vi "AlliGator Overlays Phasor Ratio or Derived Quantity on Source Image v3.vi"(7 "Image Color Scale Information":T2, 8 "Error In":errorcluster, 10 "Source Image Display":T1, 11 "AlliGator IV DVR in":refnum<data-value>) -> (0 "Error Out":errorcluster, 1 "# Overlay Pixels":i32, 2 "Source Image Display out":T1, 3 "AlliGator IV DVR out":refnum<data-value>)   [LabVIEW 2021, in "AlliGator Phasor Ratio.lvlib"]
doc: "Computes and overlays the phasor ratio map (or map of a derived quantity) on the Source Image."
uses:
  AlliGator Phasor Ratio.lvlib
  <vilib>/vision/Image Controls.llb/IMAQ Image.ctl
  AlliGator Internal Variables v2.ctl
  AlliGator Gate Image Set.ctl
  AlliGator FLI Dataset Type.ctl
  AlliGator Data Series Type.ctl
  AlliGator Dataset Channel.ctl
  AlliGator Gate Arithmetic.ctl
  AlliGator Displayed Image.ctl
  Image/Named ROI Description.ctl
  AlliGator Decay Metadata v3.ctl
  AlliGator Decay Background Subtraction Info.ctl
  AlliGator Baseline Subtraction Method.ctl
  Graphs/XY Graph/XY Graph Plot Shift Parameters.ctl
  Graphs/XY Graph/XY Graph Plot Shift Method.ctl
  AlliGator Decay Extrapolation Parameters.ctl
  Phasor/Calibration Phasor (m, phi).ctl
  Phasor/Phasor Reference Series.ctl
  Phasor/Phasor Calibration Map v2.ctl
  Phasor/Phasor (g, s).ctl
  AlliGator Raw Phasor Plot Data v4.ctl
  Phasor/Phasor Standard Deviation Options.ctl
  AlliGator Phasor Multi-Harmonic Data.ctl
  Phasor/Phasor Harmonic Data.ctl
  AlliGator Decay Fit Options & Parameters v2.ctl
  Fits/IRF(X)PSED/Decay Fit Options v2.ctl
  Fits/Decay Convolution/Decay Model.ctl
  Fits/Residual Type.ctl
  Fits/IRF(X)PSED/Fit Weights Type.ctl
  Fits/Non-linear Fitting Method v2.ctl
  Fits/Fit Calculation Method.ctl
  Fits/Non-linear Fitting Algorithm.ctl
  AlliGator Decay Fit Parameter Constraints 2.ctl
  Fits/IRF(X)PSED/Decay Fit Parameters In List.ctl
  Fits/IRF(X)PSED/MLE Baseline Offset Type.ctl
  AlliGator Decay Preprocessing Parameters.ctl
  Fits/IRF(X)PSED/Decay Fit Parameters & Derived Quantities List.ctl
  AlliGator Parameter Maps Data.ctl
  Image/Image Color Scale Information.ctl
  AlliGator Settings List.ctl
  Palette/Image Palette Information.ctl
  Image/Image Display Palette Type.ctl
  AlliGator Variables List.ctl
  AlliGator Phasor Ratio Data.ctl
  AlliGator Phasor Ratio Color-Coded Quantity.ctl
  Phasor/Phasor Ratio Type.ctl
  AlliGator Partial Data Information.ctl
  Variant/Variant to Data/Variant to DBL.vi
  Variant/Variant to Data/Variant to Boolean.vi
  Variant/Variant to Data/Variant to String.vi
  Image/Image Get Pixel Color.vi
  Image/Adjust Pixel Overlay Brightness.vi
  <vilib>/vision/NI_Vision_Development_Module.lvlib
  AlliGator Settings.lvlib
  Variant/Variant to Data/Variant to Data.lvlib
  Image/Image.lvlib
  Palette/Palette.lvlib
  AlliGator Globals, Variables & Constants.lvlib
  Time/Time.lvlib
  Error/Error.lvlib
  Phasor/Phasor.lvlib
  Utilities/Utilities.lvlib
  AlliGator Phasor Plot.lvlib
  AlliGator Decay Preprocessing.lvlib
  Graphs/XY Graph/XY Graph Add-Ons.lvlib
  AlliGator Phasor Graph.lvlib
  AlliGator Files.lvlib
  AlliGator Source Image.lvlib
  AlliGator Internal Variables.lvlib
  Fits/Fits.lvlib
  AlliGator Decay Fit.lvlib
  AlliGator Decay Fit Parameter Map.lvlib
  AlliGator Dual-Channel Datasets.lvlib
panel:
  out "Overlay Copy (s)":dbl
  out "Overlay Erase (s)":dbl
  out "Overlay Compute (s)":dbl
  # "see the AlliGator License on the block diagram (Ctrl+E or Window:Show Block Diagram)"
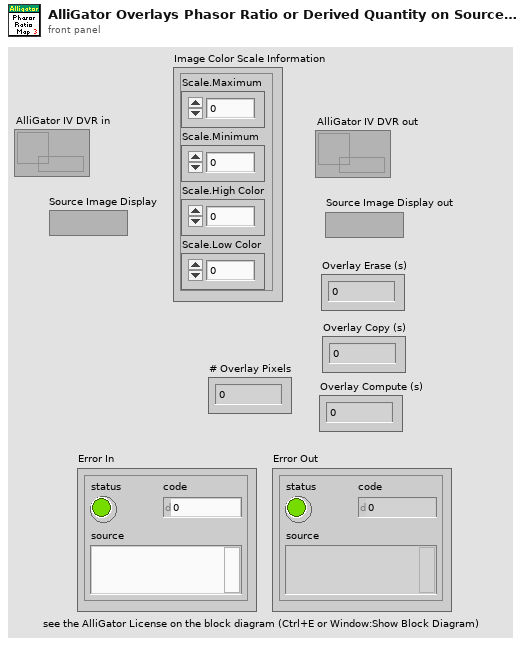
[diagram p1: front panel]
types:
  T1 = typedef "IMAQ Image.ctl" = refnum<image>
  T2 = typedef "Image.lvlib/Image Color Scale Information.ctl" = cluster{"Scale.Maximum":dbl, "Scale.Minimum":dbl, "Scale.High Color":u32, "Scale.Low Color":u32}
  T3 = typedef "AlliGator Settings.lvlib/AlliGator Settings List.ctl" = enum16{"GUI:Visible Settings Tab", "GUI:Last Run Version", "Source Image:Use Image Histogram for Contrast", "Source Image:Low Count Pixels Rejection Options", "Source Image:High Count Pixels Rejection Options", "Source Image:Use Image Brightness", "Source Image:Blend Overlay with Image Background", "Source Image:Use Fixed ROI Diameter", "Source Image:ROI Diameter", "Source Image:ROI Center Color", "Source Image:Peak Threshold", "Source Image:Intensity Threshold", "Source Image:Image Binning Options", "Source Image:Image Smoothing Options", "Source Image:Image Histogram Active", "Source Image:Invert Binary Mask", "Source Image:Hot Pixel Removal", "Source Image:Overlay Analyzed ROI Center", "Source Image:Auto-Adjust Contrast", "Source Image:Histogram Lower Percentile", "Source Image:Histogram Upper Percentile", "Source Image:Save Source Image", "Source Image:Scale Bar Options", "Source Image:Image Resolution (Pixel Size)", "Source Image:Flatfield Correction", "Source Image:Show Dead Left Columns Correction", "Source Image:Dead Left Columns Correction", "Source Image:Image Pre-Processing Operations Order", "Data Information:Gate Width", "Data Information:Nanotime Gate Separation", "Data Information:Macrotime Gate Separation", "Data Information:Gate Step", "Data Information:# Gates", "Data Information:Gate Image Exposure", "Data Information:Gate Image Integration", "Data Information:Gates to Skip", "Data Information:Gates to Keep", "Data Information:Define Gates to", "Data Information:Channel Name", "Data Information:Available Channel Names", "Data Information:Channel Arithmetic", "Data Information:Background File Subtraction", "Data Information:Background File", "Data Information:Background Scaling Factor", "Data Information:Background Pile-up Correction", "Data Information:Background Pixel Well Capacity", "Data Information:Laser Period", "Data Information:SYNC Period", "Data Information:Pile-up Correction", "Data Information:Pixel Well Capacity", "Data Information:Dataset Scaling Factor", "Fluorescence Decay_Decay Pre-Processing:Reverse Gates", "Fluorescence Decay_Decay Pre-Processing:Verbose Decay Pre-Processing", "Fluorescence Decay_Decay Pre-Processing:Use Decay Pre-Processing", "Fluorescence Decay_Decay Pre-Processing:Background Subtraction", "Fluorescence Decay_Decay Pre-Processing:Background Definition Range", "Fluorescence Decay_Decay Pre-Processing:Baseline Subtraction Method", "Fluorescence Decay_Decay Pre-Processing:Decay Pre-Processing Operations Order", "Fluorescence Decay_Decay Pre-Processing:Smoothing Parameter", "Fluorescence Decay_Decay Pre-Processing:Shift Decay", "Fluorescence Decay_Decay Pre-Processing:Decay Shift Parameters", "Fluorescence Decay_Decay Pre-Processing:Fold Decay", "Fluorescence Decay_Decay Pre-Processing:# Folds", "Fluorescence Decay_Decay Pre-Processing:1-Normalize Decay", "Fluorescence Decay_Decay Pre-Processing:[0-1]-Normalize Decay", "Fluorescence Decay_Decay Pre-Processing:Smoothen Decay", "Fluorescence Decay_Decay Pre-Processing:Extrapolate Decay", "Fluorescence Decay_Decay Pre-Processing:Use Periodicity", "Fluorescence Decay_Decay Pre-Processing:Use Cursors", "Fluorescence Decay_Decay Pre-Processing:Tail Fraction", "Fluorescence Decay_Decay Pre-Processing:Head Fraction", "Fluorescence Decay_Decay Pre-Processing:Additional Points", "Fluorescence Decay_Decay Pre-Processing:Straighten Decay", "Fluorescence Decay_Decay Pre-Processing:Constant Background", "Fluorescence Decay_Decay Pre-Processing:Pixel-Normalize Decay", "Fluorescence Decay_Advanced Analysis:Extract IRF instead of Decay", "Fluorescence Decay_Advanced Analysis:IRF Extraction Options", "Fluorescence Decay_Advanced Analysis:IRF Optimization Options", "Fluorescence Decay_Advanced Analysis:Square Pulse Options", "Fluorescence Decay_Advanced Analysis:IRF Order", "Fluorescence Decay_Advanced Analysis:IRF Time Constants", "Fluorescence Decay_Advanced Analysis:Wavelet Analysis Options", "Fluorescence Decay_Advanced Analysis:Average Lifetime Options", "Fluorescence Decay_Fit Options:Fit Options", "Fluorescence Decay_Fit Options:Use Legacy Fitting Approach", "Fluorescence Decay_Fit Options:Use Data Information Laser Period", "Fluorescence Decay_Fit Parameters:Displayed Fit Parameters", "Fluorescence Decay_Fit Parameters:Fit Parameter Constraints", "Fluorescence Decay_Fit Parameters:Export Tabulated Results", "Fluorescence Decay_Fit Parameters:MLE Baseline Offset Type", "Fluorescence Decay_Fit Parameters:MLE Baseline Offset", "Fluorescence Decay_Fit Parameters:Guess Parameter Names", "Fluorescence Decay_Fit Parameters:Guess Parameter Values", "Fluorescence Decay_Fit Parameters:Guess Parameters Options", "Fluorescence Decay_Styles:Show Last Decay Only", "Fluorescence Decay_Styles:Decay Graph Color Array", "Fluorescence Decay:Decay Graph Active", "Fluorescence Decay Statistics:Min Peak Value", "Fluorescence Decay Statistics:Reject Low Decay Peak Pixels", "Fluorescence Decay Statistics:Reject High Decay Peak Pixels", "Fluorescence Decay Statistics:Max Peak Value", "Time Traces:Use File Timestamp", "Time Traces:Time Step", "Time Traces:Use Intensity Correction File", "Time Traces:Intensity Correction File", "Phasor Plot:Phasor Plot Smoothing Options", "Phasor Plot:Phasor Plot Size", "Phasor Plot:Phasor Plot Graphics Options", "Phasor Plot:Cumulative Phasor Plot", "Phasor Plot:Use Phasor Brightness", "Phasor Plot:Blend Overlay with Phasor Background", "Phasor Plot:Save Phasor Plot", "Phasor Plot:Show References", "Phasor Plot:Phasor Ratio Decay Range", "Phasor Plot:Exponential Fading", "Phasor Plot:Phasor Ratio Reference Colors", "Phasor Plot:Reference Radius", "Phasor Plot:Show Color Map Vertices", "Phasor Plot:Phasor Plot Active", "Phasor Plot:Phasor Ratio Color Map Type", "Phasor Plot:Phasor Ratio Color Map", "Phasor Plot:Phasor Ratio Display Range", "Phasor Plot:Selected Image ROI(s)", "Phasor Plot:All Image ROIs", "Phasor Plot:Selected Phasor Plot ROI(s)", "Phasor Plot:All Phasor Plot ROIs", "Phasor Plot:Phasor Ratio Color-Coded Quantity", "Phasor Plot:Store Phasor Harmonics", "Phasor Plot:Draw Reference Segment", "Phasor Plot:User-Defined Quantity", "Phasor Graph:Phasor Frequency", "Phasor Graph:Phasor Ratio Type", "Phasor Graph:Pixel-level Phasor Computation", "Phasor Graph:Save Phasor Graph", "Phasor Graph:Phasor Graph Active", "Phasor Graph:Phasor SDV Options", "Phasor Calibration:Use Backup Calibration if needed", "Phasor Graph:Define Shortest Lifetime as", "Phasor Calibration:Backup Calibration Type", "Phasor Calibration:Calibration Type", "Phasor Calibration:Calibration Lifetime", "Phasor Calibration:Calibration Map Algorithm", "Single-Exponential Phasor Locus (SEPL):Gate Parameters", "Single-Exponential Phasor Locus (SEPL):User-defined Gate", "Single-Exponential Phasor Locus (SEPL):User-defined IRF", "Single-Exponential Phasor Locus (SEPL):Phasor Parameters", "Single-Exponential Phasor Locus (SEPL):Decay & IRF Parameters", "Single-Exponential Phasor Locus (SEPL):Display Parameters", "Lifetime Analysis:Decay Analysis Parameters", "Lifetime Analysis:Lifetime Map Active", "Plugins:Python Settings", "Miscellaneous:Verbose Mode", "Miscellaneous:Beep after Script", "Miscellaneous:Saved Image File Format", "Miscellaneous:Exported Gate Image Settings", "Miscellaneous:Include Loading in Timing", "Miscellaneous:Verbose Settings Mode", "Miscellaneous:Histogram Options", "Miscellaneous:Beep on Error", "Miscellaneous:# Logical Processors Used", "Miscellaneous:ROI Description Max Characters", "Miscellaneous:Verbose Error Mode", "Miscellaneous:Transparent Mask Color"}
  T4 = typedef "AlliGator Settings.lvlib/AlliGator Partial Data Information.ctl" = cluster{"Laser Period":dbl[unit], "SYNC Period":dbl[unit], "# Gates":u32, "Gate Separation":dbl[unit]}
  T5 = typedef "Phasor.lvlib/Phasor Ratio Type.ctl" = enum32{"Intensity-weighted", "Amplitude-weighted"}
  T6 = typedef "AlliGator Phasor Ratio.lvlib/AlliGator Phasor Ratio Color-Coded Quantity.ctl" = enum16{"Phasor Ratio (f1 or a1)", "Average Lifetime (<tau>_i or <tau>_a))", "User-Defined Quantity"}
  T7 = typedef "AlliGator Phasor Ratio.lvlib/AlliGator Phasor Ratio Data.ctl" = cluster{"Complex Phasor":csg, "Phasor Ratio":sgl, "z_1":csg, "z_2":csg, "Mapped Quantity":sgl}
  T8 = typedef "AlliGator Globals, Variables & Constants.lvlib/AlliGator Variables List.ctl" = enum16{"---- GUI ----", "GUI:Initialization Status", "GUI:State Indicators Refnum", "GUI:Original AlliGator Menu Items", "GUI:Current Action Loop State", "GUI:Script in progress", "GUI:Playback", "GUI:Loop Playback", "GUI:Search ROI Used", "GUI:Search ROI", "Decay Graph Max Legend Size", "Intensity Graph Max Legend Size", "Decay Statistics Graph Max Legend Size", "Phasor Graph Max Legend Size", "Phasor Ratio Graph Max Legend Size", "Lifetime Graph Max Legend Size", "---- Files ----", "Files:Export Dataset Frames as Individual Files", "Files:Show Batch Export Help Balloons", "Files:Frames in Dataset", "Files:ptu File Frame Start Indices", "Files:Current Frame in Dataset", "Files:Current Frame Timestamp", "Files:Dataset Loaded", "Files:Dataset Metadata", "Files:Dataset Channel", "Files:Dataset Data Description", "Files:Background Dataset Metadata", "Files:Background Dataset Channel", "Files:Background Dataset Data Description", "Files:Background File Subtraction", "Files:Background File Path", "Files:Background File Pile-up Correction", "Files:Background File Pixel Well Capacity", "Files:Background File Scaling Factor", "Files:Current Dataset Load Settings", "Files:Dataset Path", "Files:ICCD-specific Information", "Files:Macrotime Gate Separation", "------ Python Plugins ------", "Python Plugins:Information", "Python Plugins:Python Session", "Python Plugins:Valid Python Session?", "---- Source Image ----", "Source Image:ROIs", "Source Image:Current ROI", "Source Image:ROI Event Refnum", "X_Source Image Display Range", "X_Source Image Palette Information", "X_Type of Displayed Image", "X_Time Gate Slider", "Source Image:Palette List", "Source Image:Scale", "Source Image:ROI Overlay Color", "Source Image:Overlay to Erase", "Source Image:Is Displayed Image Accumulated", "Source Image:White Light Image Modified", "Source Image:Mask Image Modified", "---- Image Profile Window ----", "Image Profile:Overlay ROI in Source Image", "Image Profile:Window Event Refnum", "Image Profile:IntensityType", "Image Profile:Intensity Average Type", "Image Profile:Intensity-weighted SDV", "Image Profile:Box Profile Type", "Image Profile:Window Open", "Image Profile:Plotted Fit Parameter", "------ Phasor Graph -------", "Phasor Graph:Show Line", "---- Phasor Plot ---", "Phasor Plot:Parameters Changed", "Phasor Plot:FLI Dataset Modified since last Calculation", "Phasor Harmonics Data", "Selected Phasor Harmonics", "Phasor Harmonic Manager Event Refnum", "Phasor Plot:ROIs", "Phasor Plot:Current ROI", "Phasor Plot:ROI Event Refnum", "Phasor Plot:Image Reference Points", "Phasor Plot:Computed", "Phasor Plot:Palette Information", "Phasor Plot:Palette List", "Phasor Plot:Phasor Ratio Palette Information", "Phasor Plot:Phasor Ratio Palette List", "Phasor Plot:Image Scale", "Phasor Plot:Image Overlay to Erase", "Phasor Plot:Image Elements to Update", "Phasor Plot:Current Calculation Parameters", "Phasor Plot:Current Calibration Options", "Phasor Plot:Reset Cumulated Phasor Plot", "Phasor Plot:Reference 1", "Phasor Plot:Lifetime Reference 1", "Phasor Plot:Reference 1 Frequency", "Phasor Plot:Reference 2", "Phasor Plot:Lifetime Reference 2", "Phasor Plot:Reference 2 Frequency", "---- Decay Analysis ----", "Number of Selected Decays to Fit", "LS Fit Results", "LAR Fit Results", "BS Fit Results", "Last Decay Max - Min", "Best Fit Parameters", "Best Fit Parameter Names", "Actual Size X", "Actual Size Y", "Binning X", "Binning Y", "Actual # Gates", "Dataset Number", "Gates to...", "Gates Skipped", "Gates to keep", "Gate Step", "Gate Separation", "Reversed Gates", "Pile-up Correction", "Pixel Well Capacity", "Background Subtracted", "Background Subtraction Method", "Background Definition Range", "Background File (deprecated)", "Number of Dataset Accumulated", "Array of Accumulated Dataset Paths", "Do Averaged Datasets", "Destination File Path", "Process Plot Target", "Use 1/D as Phasor Frequency", "---- Decay Fit Parameter Map -----", "Decay Fit Parameter Map:Palette Information", "Decay Fit Parameter Map:Palette List", "------- Local Decay Window ---------", "Local Decay Graph Window:Event Refnum", "Local Decay Graph Window:Use normalized IRF for convolution", "----- Miscellaneous ----", "Misc:Skippable Dialog Windows Status"}
  T9 = typedef "Palette.lvlib/Image Palette Information.ctl" = cluster{"Palette Name [# Colors,int?,inv?]":string, "Palette Type":T10, "Palette Colors":u32[], "Interpolate?":bool}
  T10 = typedef "Image.lvlib/Image Display Palette Type.ctl" = u32
  T11 = enum32{"Interpolate Reference Colors", "Use Custom Map"}
  T12 = cluster{"Reference 1":u32, "Reference 2":u32, "Boundary":u32}
  T13 = typedef "Phasor.lvlib/Phasor (g, s).ctl" = cluster{"g":dbl, "s":dbl}
  T14 = typedef "AlliGator Internal Variables.lvlib/AlliGator Internal Variables v2.ctl" = cluster{"Displayed Image":T1, "White Light Image":T1, "Mask Image":T1, "ROI Mask Image":T1, "Current Dataset Images 1":T15, "Background Dataset Images 1":T15, "Current Dataset Images 2":T15, "Background Dataset Images 2":T15, "Current Dataset Arithmetic Images":T15, "Accumulated Dataset Images 1":T15, "Accumulated Dataset Images 2":T15, "Accumulated Dataset Arithmetic Images":T15, "Phasor Plot Image":T1, "Decay Fit Parameter Map Image":T1, "Single Data Point Path":path, "White Light Image Path":path, "Mask Image Path":path, "Time-Series Folder":path, "[Time-Series Paths]":path[], "Current Dataset":i32, "Single Dataset Type":T16, "Current Folder":string, "AlliGator Data Series Type":T17, "# Datasets":i32, "Dual-Channel Dataset":bool, "Selected Channel Name":string, "Dataset Channel":T18, "Channel Arithmetic":T19, "Dual-Channel Background Dataset":bool, "Background Channel":T18, "Dual-Channel Accumulated Dataset":bool, "Start Time":dbl, "[Time-Series Timestamps]":dbl[], "[Intensity Corrections]":dbl[], "Time Series Script":bool, "Type of Displayed Image":T20, "Gate Image Slide":u16, "# Gates":i32, "ROIs":T21[], "ROI Decay":cluster{"t Array":dbl[], "I Array":dbl[]}, "Valid Decay":bool, "Decay  Metadata":T23, "Reference Decay Plot Name":string, "Reference Decay":cluster{"t Array":dbl[], "I Array":dbl[]}, "Decay Shift Plot":cluster{"Time Stamps":dbl[], "Decay Shifts":dbl[]}, "[Decays Max Values]":sgl[], "[Decays Min Values]":sgl[], "Calibration Phasor":T29, "Calibration Phasor Series":T30, "Phasor Calibration Map":T31, "Calibration Map MD5 Digest":string, "Last Raw Phasor":T13, "Last Calibrated Phasor":T13, "Last Calibrated Phasor SDV":T13, "Phasor Graph:Phasor Plot":cluster{"g Array":dbl[], "s Array":dbl[]}, "Phasor Graph:Phasor SDV Plot":cluster{"g Array":dbl[], "s Array":dbl[]}, "[Phasor Graph:Raw Phasor Plots]":T32[], "Phasor Plot locked to Ref 1":i32, "[Phasor Plot(s) locked to Ref 1]":i32[], "[Phasor Plot(s) locked to Ref 2]":i32[], "[Pixel Phasors]":T13[], "[[Sum Image]]":dbl[][], "[[CSG Phasors]]":csg[][], "[[Valid Pixel?]]":bool[][], "I/m/phi Dataset":cluster{"I/m/phi Dataset?":bool, "Base Frequency":dbl[unit], "Harmonic Orders":u8[]}, "Multi Phasor Plot Data":T34, "Decay Fit Options & Parameters":T36, "Fit Options: Decay Preprocessing Parameters":T47, "Fit Options: Reference Decay":cluster{"t Array":dbl[], "I Array":dbl[]}, "Is Full Image Parameters Map":bool, "Is Single-Pixels Parameters Map":bool, "NLSF Parameters Map X Resolution":i32, "NLSF Parameters Map Y Resolution":i32, "[Single Decay Fit Parameters]":dbl[], "Fit Model":T38, "[[Multiple Decays Fit Parameters]]":dbl[][], "[[Multiple Decays Fit Parameter SDVs]]":dbl[][], "[[IRFs]]":dbl[][], "IRF Array Time Axis":dbl[], "Decay Array Time Axis":dbl[], "[Decay Fit Parameter Names]":T48[], "[[Phasor Ratios]]":dbl[][], "[[Average Lifetimes]]":dbl[][], "Amplitude Weighted Average Lifetime":bool, "[Decay Sum]":dbl[], "Parameter Maps":T49[], "[[User-defined Quantities]]":dbl[][], "User-defined Quantity":string}
  T15 = typedef "AlliGator Internal Variables.lvlib/AlliGator Gate Image Set.ctl" = cluster{"SGL Image Max":T1, "SGL Image Sum":T1, "SGL Gate Images":T1[], "SGL Image Min":T1}
  T16 = typedef "AlliGator Files.lvlib/AlliGator FLI Dataset Type.ctl" = enum16{"HDF5 FLI Dataset", "Gate Image Folder", ".sdt FLI Dataset (Becker & Hickl)", ".ptu FLI Dataset (PicoQuant)", "SS1 FLI Dataset", "SS2 FLI Dataset", "I/m/phi Dataset", ".bin FLI Dataset (PicoQuant Binned)", ".bin FLI Dataset (Piccolo Binned)"}
  T17 = typedef "AlliGator Files.lvlib/AlliGator Data Series Type.ctl" = enum16{"Not a Supported Series", "Gate Images Folder Series", "SwissSPAD 2 Dataset Series", "B&H FLI Dataset Series", "PicoQuant PTU FLI Dataset Series", "PicoQuant BIN FLI Dataset Series", "Piccolo hist BIN FLI Dataset Series", "HDF5 FLI Dataset Series"}
  T18 = typedef "AlliGator Dual-Channel Datasets.lvlib/AlliGator Dataset Channel.ctl" = enum16{"G2", "INT"}
  T19 = typedef "AlliGator Settings.lvlib/AlliGator Gate Arithmetic.ctl" = enum16{"None", "INT-G2", "G2/INT*<INT>", "(1 - G2/INT)*<INT>"}
  T20 = typedef "AlliGator Source Image.lvlib/AlliGator Displayed Image.ctl" = enum16{"Single Gate", "Sum of All Gates", "Max of All Gates", "Min of All Gates", "-", "White Ligth Image", "Mask Image"}
  T21 = typedef "Image.lvlib/Named ROI Description.ctl" = cluster{"ROI Descriptor":T22, "ROI Name":string, "Overlay Color":u32}
  T22 = typedef "ROI Descriptor" = cluster{"Global Rectangle":i32[], "Contours":cluster{"ID":enum32{"External", "Internal"}, "Type":u32, "Coordinates":i32[]}[]}
  T23 = typedef "AlliGator Phasor Graph.lvlib/AlliGator Decay Metadata v3.ctl" = cluster{"ROI Descriptor":T22, "ROI Center":cluster{"X":i32, "Y":i32}, "Decay Background Subtraction Info":T24, "Decay Reverted":bool, "Decay Smoothened":bool, "Decay Straightened":bool, "Fitted Tau (Decay Straightening)":dbl, "Decay Shift Parameters":T26, "Decay Shifted":bool, "Decay Extrapolated":bool, "Decay Extrapolation Parameters":T28, "Decay Normalized":bool, "Fold Decay":bool, "# Folds":u32}
  T24 = typedef "AlliGator Decay Analysis.lvlib/AlliGator Decay Preprocessing.lvlib/AlliGator Decay Background Subtraction Info.ctl" = cluster{"Laser Period":dbl[unit], "Gate Duration":dbl[unit], "Baseline Subtraction Method":T25, "Background Definition Range":cluster{"Min Gate":dbl[unit], "Max Gate":dbl[unit]}, "Total Intensity w/o Bkgd Subtraction":dbl, "Bkgd-subtracted Intensity (exp)":dbl, "# Data Points":i32, "Background/Gate":dbl, "Fitted Lifetime":dbl[unit], "Bkgd-subtracted Intensity (theo)":dbl}
  T25 = typedef "AlliGator Decay Analysis.lvlib/AlliGator Decay Preprocessing.lvlib/AlliGator Baseline Subtraction Method.ctl" = enum16{"Mean", "Min", "Square Gated Single-Exponential", "File", "Constant"}
  T26 = typedef "XY Graph Add-Ons.lvlib/XY Graph Plot Shift Parameters.ctl" = cluster{"Type":T27, "Shift":dbl[unit], "Threshold":dbl, "Rotate":bool}
  T27 = typedef "XY Graph Add-Ons.lvlib/XY Graph Plot Shift Method.ctl" = enum16{"Default", "CFD", "Threshold", "Cross-Correlation"}
  T28 = typedef "AlliGator Decay Analysis.lvlib/AlliGator Decay Preprocessing.lvlib/AlliGator Decay Extrapolation Parameters.ctl" = cluster{"Additional Points":u32, "Head Fraction":dbl, "Fitted Tau":dbl, "Use Periodicity":bool, "Use Cursors":bool, "Tail Fraction":dbl}
  T29 = typedef "Phasor.lvlib/Calibration Phasor (m, phi).ctl" = cluster{"m":dbl, "phi":dbl, "Phasor Frequency":dbl[unit], "Reference Lifetime":dbl[unit]}
  T30 = typedef "Phasor.lvlib/Phasor Reference Series.ctl" = cluster{"m Array":dbl[], "phi Array":dbl[], "Phasor Frequency":dbl[unit], "Calibration Lifetime":dbl[unit]}
  T31 = typedef "Phasor.lvlib/Phasor Calibration Map v2.ctl" = cluster{"Phasor Frequency":dbl[unit], "Calibration Lifetime":dbl[unit], "ROI Centers":cluster{"X":i32, "Y":i32}[], "ROI Descriptors":T22[], "Map Resolution X":i32, "Map Resolution Y":i32, "z Array":cdb[]}
  T32 = typedef "AlliGator Phasor Graph.lvlib/AlliGator Raw Phasor Plot Data v4.ctl" = cluster{"Phasor Plot Name":string, "Raw Phasor Plot":T13[], "Phasor Frequency":dbl[unit], "[Decay Metadata]":T23[], "Raw Phasor Plot SDV":T13[], "Phasor SDV Options":T33, "[Calibration Phasor]":T29[]}
  T33 = typedef "Phasor.lvlib/Phasor Standard Deviation Options.ctl" = cluster{"Compute Estimated SDV":bool, "# Replicas":u32, "Use Estimated Average Phasor":bool}
  T34 = typedef "AlliGator Phasor Plot.lvlib/AlliGator Phasor Multi-Harmonic Data.ctl" = cluster{"Base Frequency":dbl[unit], "# Harmonics":u8, "Harmonic Orders":u8[], "Phasor Plot Settings Checksum":u64, "Phasor Harmonic Data Array":T35[]}
  T35 = typedef "Phasor.lvlib/Phasor Harmonic Data.ctl" = cluster{"Phasor Harmonic Name":string, "Phasor Plot Settings Checksum":u64, "Phasor Frequency":dbl[unit], "Base Frequency":dbl[unit], "Harmonic Order":u8, "Phasor Plot Parameters":string, "Phasor Array [[CSG]]":csg[][], "Dataset File Path":path}
  T36 = typedef "AlliGator Decay Fit Parameter Map.lvlib/AlliGator Decay Fit Options & Parameters v2.ctl" = cluster{"SYNC Period":dbl[unit], "Fit Options":T37, "Fit Parameter Constraints":T44[], "MLE Baseline Offset":dbl, "MLE Baseline Offset Type":T46}
  T37 = typedef "Fits.lvlib/Decay Fit Options v2.ctl" = cluster{"Show Fit Residuals":bool, "Fit Model":T38, "Residual Type":T39, "Max Decay Percentile":dbl, "Min Decay Percentile":dbl, "Show Full Decay":bool, "Weights":T40, "Fitting Method":T41, "Compute Parameter Uncertainties":bool, "Periodic Boundaries":bool, "Model Calculation":T42, "Period":dbl[unit], "Termination Criteria":cluster{"Max Iterations":i32, "Max Function Calls":i32, "Max Time":dbl[unit], "Function Tolerance":dbl, "Parameter Tolerance":dbl, "Gradient Tolerance":dbl, "Min Lambda":dbl, "Max Lambda":dbl, "Initial Tick Count":u32}, "Offset Resolution":dbl[unit], "Use Local IRF":bool, "Fitting Algorithm":T43}
  T38 = typedef "Fits.lvlib/Decay Model.ctl" = enum16{"1-Exponential", "2-Exponentials"}
  T39 = typedef "Fits.lvlib/Residual Type.ctl" = enum16{"Standard", "Normalized", "Reduced"}
  T40 = typedef "Fits.lvlib/Fit Weights Type.ctl" = enum16{"Unweighted", "1/Variance", "Best of All"}
  T41 = typedef "Fits.lvlib/Non-linear Fitting Method v2.ctl" = enum16{"Least Square", "Least Absolute Residual", "Bisquare", "MLE", "-", "Best of All"}
  T42 = typedef "Fits.lvlib/Fit Calculation Method.ctl" = enum16{"Simulation", "Convolution", "Integration"}
  T43 = typedef "Fits.lvlib/Non-linear Fitting Algorithm.ctl" = enum16{"Levenberg-Marquardt", "Trust-Region Dogleg"}
  T44 = typedef "AlliGator Decay Analysis.lvlib/AlliGator Decay Fit.lvlib/AlliGator Decay Fit Parameter Constraints 2.ctl" = cluster{"Fit Parameter":T45, "Min Value":dbl, "Max Value":dbl, "Global":bool, "Used":bool}
  T45 = typedef "Fits.lvlib/Decay Fit Parameters In List.ctl" = enum16{"Offset", "Baseline", "A_1", "tau_1", "A_2", "tau_2"}
  T46 = typedef "Fits.lvlib/MLE Baseline Offset Type.ctl" = enum32{"Absolute", "Percentage"}
  T47 = typedef "AlliGator Decay Analysis.lvlib/AlliGator Decay Preprocessing.lvlib/AlliGator Decay Preprocessing Parameters.ctl" = cluster{"Background Subtraction":bool, "Straighten Decay":bool, "Reverse Gates":bool, "1-Normalized Decay":bool, "Smoothen Decay":bool, "Smoothing Parameter":dbl, "Shift Decay":bool, "Decay Shift Parameters":T26, "Extrapolate Decay":bool, "Additional Points":u32, "Head Fraction":dbl, "Pixel-Normalize Decay":bool, "Use Periodicity":bool, "Use Cursors":bool, "Tail Fraction":dbl, "Use Decay Pre-Processing":bool, "Fold Decay":bool, "# Folds":u32, "[0-1]-Normalized Decay":bool}
  T48 = typedef "Fits.lvlib/Decay Fit Parameters & Derived Quantities List.ctl" = enum16{"Offset", "Baseline", "A_1", "tau_1", "A_2", "tau_2", "<tau>_a", "f1_a", "f2_a", "<tau>_i", "f1_i", "f2_i", "-", "R^2", "Chi^2"}
  T49 = typedef "AlliGator Parameter Maps Data.ctl" = cluster{"Map Set Name":string, "[Parameter Names]":string[], "[[Parameters]]":dbl[][], "[[Parameter SDVs]]":dbl[][], "Decay Array Time Axis":dbl[], "[[IRFs]]":dbl[][], "IRF Array Time Axis":dbl[]}
  T50 = cluster{"Red (or Hue) value":u8, "Green (or Sat) value":u8, "Blue (or Light or Val) value":u8}
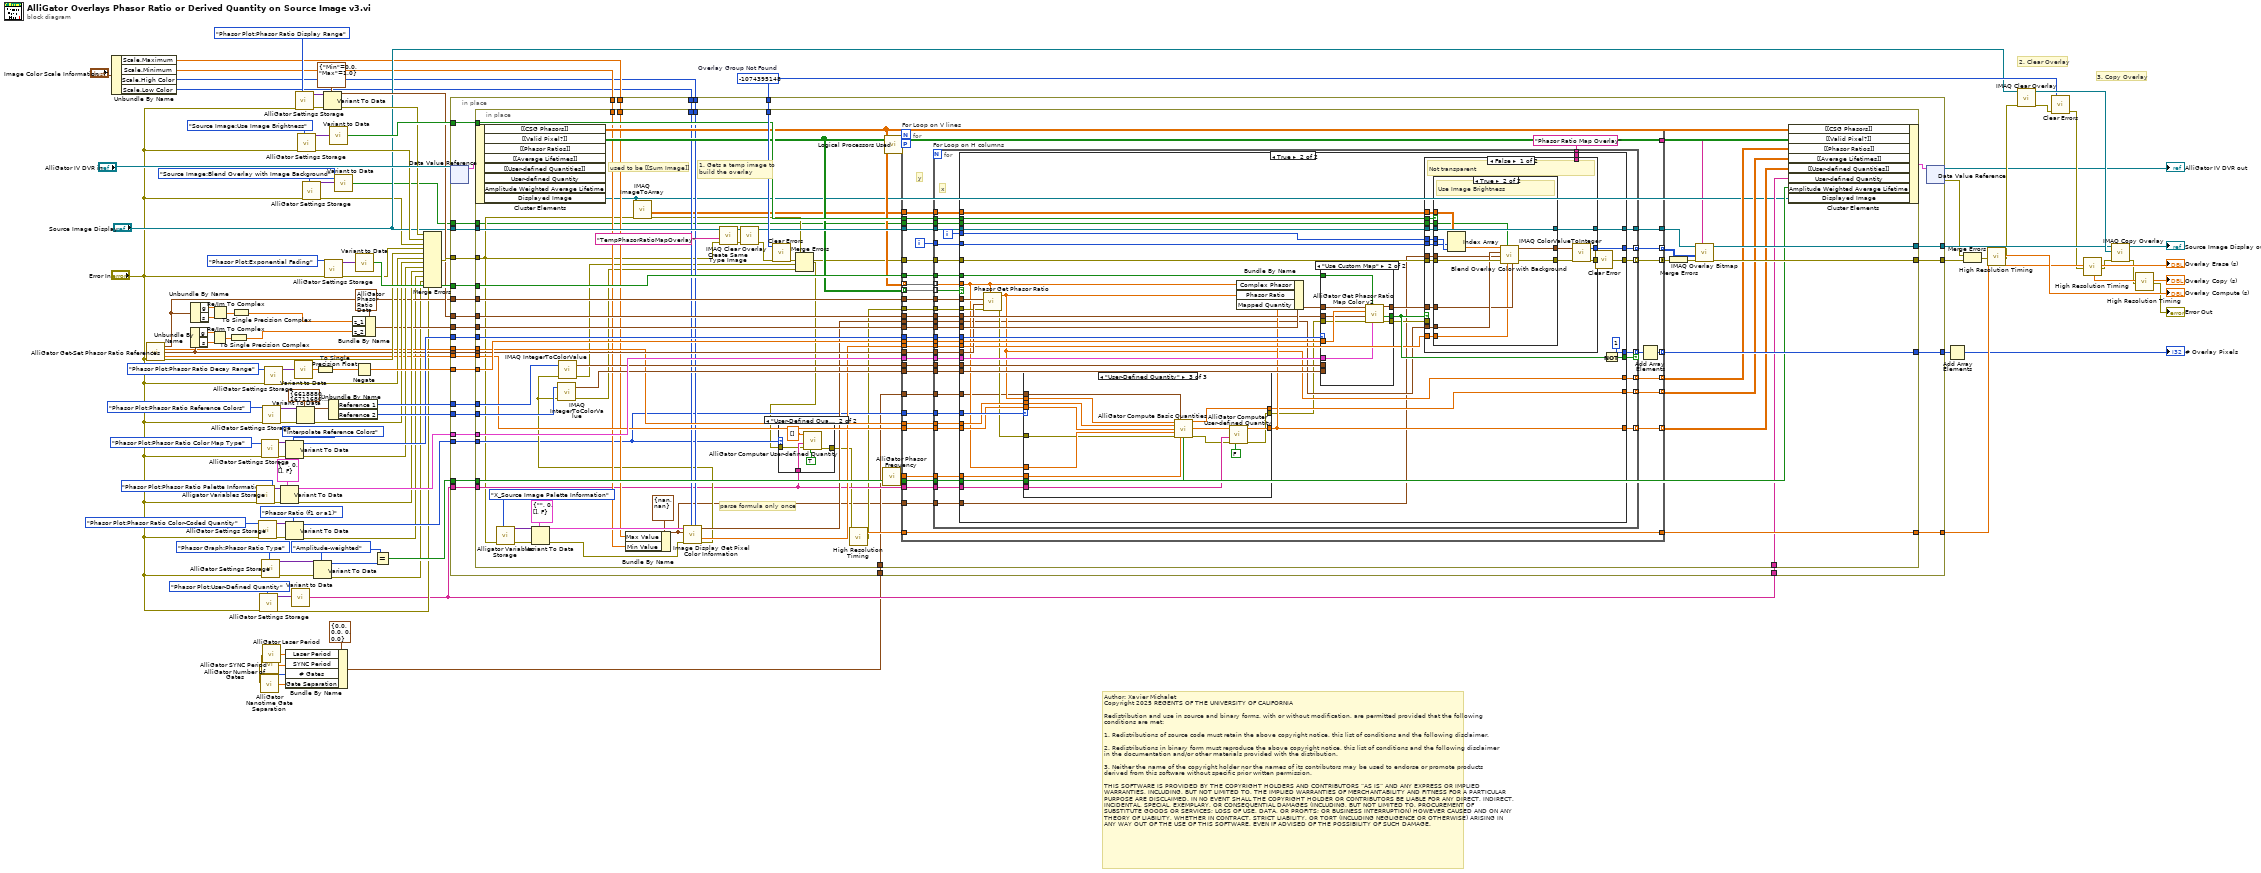
[diagram p0: block diagram]
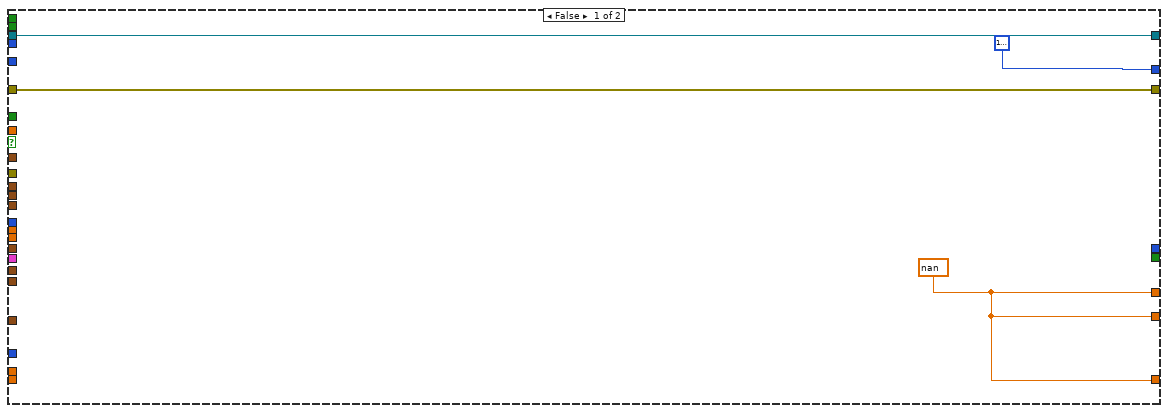
[diagram p2: hidden frame]
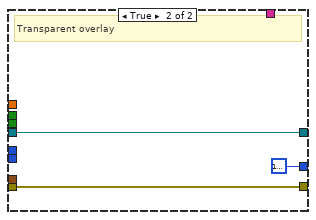
[diagram p4: hidden frame]
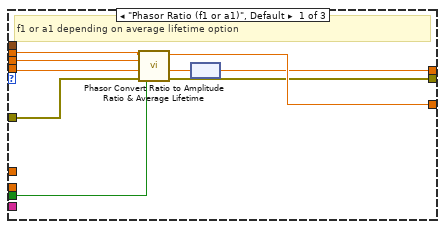
[diagram p5: hidden frame]
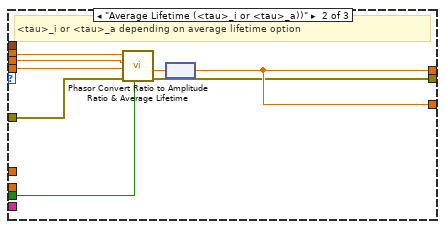
[diagram p6: hidden frame]
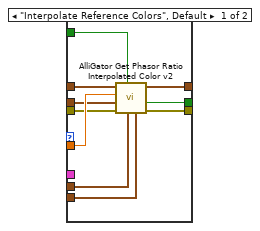
[diagram p7: hidden frame]
diagram:
  w28 = Phasor_Ratio_Type."Amplitude-weighted" ("Phasor Ratio Type")
  w88 = -1074395148  # Overlay Group Not Found
  # "Author: Xavier Michalet\nCopyright 2025 REGENTS OF THE UNIVERSITY OF CALIFORNIA\n\nRedistribution and use in source and binary forms, with or without modification, are permitted provided that the following conditions are met:\n\n1. Redistributions of source code must retain the above copyright notice, this list of conditions and the following disclaimer.\n\n2. Redistributions in binary form must reproduce the above copyright notice, this list of conditions and the following disclaimer in the documentation and/or other materials provided with the distribution.\n\n3. Neither the name of the copyright holder nor the names of its contributors may be used to endorse or promote products derived from this software without specific prior written permission.\n\nTHIS SOFTWARE IS PROVIDED BY THE COPYRIGHT HOLDERS AND CONTRIBUTORS “AS IS” AND ANY EXPRESS OR IMPLIED WARRANTIES, INCLUDING, BUT NOT LIMITED TO, THE IMPLIED WARRANTIES OF MERCHANTABILITY AND FITNESS FOR A PARTICULAR PURPOSE ARE DISCLAIMED. IN NO EVENT SHALL THE COPYRIGHT HOLDER OR CONTRIBUTORS BE LIABLE FOR ANY DIRECT, INDIRECT, INCIDENTAL, SPECIAL, EXEMPLARY, OR CONSEQUENTIAL DAMAGES (INCLUDING, BUT NOT LIMITED TO, PROCUREMENT OF SUBSTITUTE GOODS OR SERVICES; LOSS OF USE, DATA, OR PROFITS; OR BUSINESS INTERRUPTION) HOWEVER CAUSED AND ON ANY THEORY OF LIABILITY, WHETHER IN CONTRACT, STRICT LIABILITY, OR TORT (INCLUDING NEGLIGENCE OR OTHERWISE) ARISING IN ANY WAY OUT OF THE USE OF THIS SOFTWARE, EVEN IF ADVISED OF THE POSSIBILITY OF SUCH DAMAGE."
  # "3. Copy Overlay"
  # "2. Clear Overlay"
  n1 = Unbundle By Name("Image Color Scale Information") -> ("Scale.Maximum"=w20:dbl, "Scale.Minimum"=w19:dbl, "Scale.High Color"=w18:u32, "Scale.Low Color"=w17:u32)
  n2 = call "AlliGator Get-Set Phasor Ratio References.vi"("error in (no error)"="Error In") -> ("Reference Phasor 1"=w36:T13, "Reference Lifetime 1"=w32:dbl[unit], "Reference Phasor 2"=w35:T13, "Reference Lifetime 2"=w31:dbl[unit], "error out"=w71:errorcluster)  [unwired: 7 in, 3 out]
  n3 = Unbundle By Name(w35) -> ("g"=w104:dbl, "s"=w105:dbl)
  n4 = Unbundle By Name(w36) -> ("g"=w113:dbl, "s"=w112:dbl)
  n5 = Re/Im To Complex(1:w105, 2:w104) -> (0:w106:cdb)
  n6 = Re/Im To Complex(1:w112, 2:w113) -> (0:w111:cdb)
  n7 = To Single Precision Complex(1:w106) -> (0:w34:csg)
  n8 = To Single Precision Complex(1:w111) -> (0:w42:csg)
  n9 = call "Alligator Variables Storage.vi"("AlliGator Variable"=AlliGator_Variables_List."Phasor Plot:Phasor Ratio Palette Information" ("Alligator Variable"), "Error In"="Error In") -> ("Error Out"=w76:errorcluster, "Data out"=w77:variant)  [unwired: 7 in, 1 out]
  n10 = call "AlliGator Settings Storage.vi"("AlliGator Settings List"=AlliGator_Settings_List."Phasor Plot:Phasor Ratio Color-Coded Quantity", "Error In"="Error In") -> ("Error Out"=w40:errorcluster, "Variant Data out"=w39:variant)  [unwired: 8 in]
  n11 = call "AlliGator Settings Storage.vi"("AlliGator Settings List"=AlliGator_Settings_List."Phasor Plot:User-Defined Quantity", "Error In"="Error In") -> ("Error Out"=w14:errorcluster, "Variant Data out"=w15:variant)  [unwired: 8 in]
  n12 = call "AlliGator Number of Gates.vi"() -> ("# Gates"=w6:u32)
  n13 = call "AlliGator Nanotime Gate Separation.vi"() -> ("Nanotime Gate Separation"=w8:dbl[unit])
  n14 = call "AlliGator Settings Storage.vi"("AlliGator Settings List"=AlliGator_Settings_List."Phasor Plot:Phasor Ratio Color Map Type", "Error In"="Error In") -> ("Error Out"=w81:errorcluster, "Variant Data out"=w82:variant)  [unwired: 8 in]
  n15 = call "AlliGator SYNC Period.vi"() -> ("SYNC Period"=w9:dbl[unit])
  n16 = call "AlliGator Settings Storage.vi"("AlliGator Settings List"=AlliGator_Settings_List."Phasor Graph:Phasor Ratio Type", "Error In"="Error In") -> ("Error Out"=w26:errorcluster, "Variant Data out"=w27:variant)  [unwired: 8 in]
  n17 = call "AlliGator Laser Period.vi"() -> ("Laser Period"=w10:dbl[unit])
  n18 = call "AlliGator Settings Storage.vi"("AlliGator Settings List"=AlliGator_Settings_List."Phasor Plot:Phasor Ratio Reference Colors", "Error In"="Error In") -> ("Error Out"=w83:errorcluster, "Variant Data out"=w101:variant)  [unwired: 8 in]
  n19 = call "AlliGator Settings Storage.vi"("AlliGator Settings List"=AlliGator_Settings_List."Phasor Plot:Phasor Ratio Decay Range", "Error In"="Error In") -> ("Error Out"=w70:errorcluster, "Variant Data out"=w109:variant)  [unwired: 8 in]
  n20 = Variant To Data(error in=w76, type=T9 {"Palette Name [# Colors,int?,inv?]"="", "Palette Type"=0, "Palette Colors"=[], "Interpolate?"=FALSE} ("Image Display Palette Information"), Variant=w77) -> (data=w74:T9, error out=w67:errorcluster)
  n21 = Variant To Data(error in=w81, type=T11."Interpolate Reference Colors" ("Phasor Ratio Color Map Type"), Variant=w82) -> (data=w79:T11, error out=w68:errorcluster)
  n22 = Variant To Data(error in=w40, type=AlliGator_Phasor_Ratio_Color-Coded_Quantity."Phasor Ratio (f1 or a1)" ("Displayed Quantity"), Variant=w39) -> (data=w33:T6, error out=w24:errorcluster)
  n23 = Bundle By Name(cluster=T4 {"Laser Period"=0.0, "SYNC Period"=0.0, "# Gates"=0, "Gate Separation"=0.0} ("Data Information"), "Laser Period"=w10, "SYNC Period"=w9, "# Gates"=w6, "Gate Separation"=w8) -> (w7:T4)
  n24 = call-poly "Variant to Data.vi"("Variant"=w15) -> ("String"=w12:string)  [unwired: 8 in]
  n25 = call-poly "Variant to Data.vi"("Variant"=w109) -> ("Value"=w108:dbl)  [unwired: 8 in]
  n26 = call "AlliGator Settings Storage.vi"("AlliGator Settings List"=AlliGator_Settings_List."Phasor Plot:Phasor Ratio Display Range", "Error In"="Error In") -> ("Error Out"=w48:errorcluster, "Variant Data out"=w46:variant)  [unwired: 8 in]
  n27 = Variant To Data(error in=w83, type=T12 {"Reference 1"=6618880, "Reference 2"=16711680, "Boundary"=16776960} ("Phasor Ratio Reference Colors"), Variant=w101) -> (data=w99:T12, error out=w69:errorcluster)
  n28 = call "AlliGator Settings Storage.vi"("AlliGator Settings List"=AlliGator_Settings_List."Source Image:Use Image Brightness", "Error In"="Error In") -> ("Error Out"=w50:errorcluster, "Variant Data out"=w87:variant)  [unwired: 8 in]
  n29 = call "AlliGator Settings Storage.vi"("AlliGator Settings List"=AlliGator_Settings_List."Source Image:Blend Overlay with Image Background", "Error In"="Error In") -> ("Error Out"=w2:errorcluster, "Variant Data out"=w5:variant)  [unwired: 8 in]
  n30 = Variant To Data(error in=w26, type=w28, Variant=w27) -> (data=w29:T5, error out=w13:errorcluster)
  n31 = To Single Precision Float(number=w108) -> (single precision float=w107:sgl)
  n32 = Variant To Data(error in=w48, type=cluster{"Min":dbl, "Max":dbl} {"Min"=0.0, "Max"=1.0} ("Phasor Ratio Display Range"), Variant=w46) -> (data=w37:cluster{"Min":dbl, "Max":dbl}, error out=w47:errorcluster)
  n33 = call "AlliGator Settings Storage.vi"("AlliGator Settings List"=AlliGator_Settings_List."Phasor Plot:Exponential Fading", "Error In"="Error In") -> ("Error Out"=w72:errorcluster, "Variant Data out"=w95:variant)  [unwired: 8 in]
  n34 = Unbundle By Name(w99) -> ("Reference 1"=w98:u32, "Reference 2"=w97:u32)
  n35 = call-poly "Variant to Data.vi"("Variant"=w87) -> ("Value"=w85:bool)  [unwired: 8 in]
  n36 = call-poly "Variant to Data.vi"("Variant"=w5) -> ("Value"=w1:bool)  [unwired: 8 in]
  n37 = Bundle By Name(cluster=T7 {"Complex Phasor"=0.0+0.0i, "Phasor Ratio"=0.0, "z_1"=0.0+0.0i, "z_2"=0.0+0.0i, "Mapped Quantity"=0.0} ("Phasor Ratio Data"), "z_1"=w42, "z_2"=w34) -> (w43:T7)
  n38 = Negate(x=w107) -> (-x=w103:sgl)
  n39 = call-poly "Variant to Data.vi"("Variant"=w95) -> ("Value"=w94:bool)  [unwired: 8 in]
  n40 = Equal?(x=w28, y=w29) -> (x = y?=w25:bool)
  n41 = Merge Errors(w47, w50, w2, w72, w71, w70, w69, w68, w67, w24, w13, w14) -> (w73:errorcluster)
  n42 = in-place {
    in-place-border: w103 -> [w145]
    in-place-border: w98 -> [w144]
    in-place-border: w97 -> [w143]
    in-place-border: w94 -> [w142]
    in-place-border: [w141] -> w93
    in-place-border: [w140] -> w90
    in-place-border: "Source Image Display" -> [w139]
    in-place-border: w88 -> [w138]
    in-place-border: w85 -> [w137]
    in-place-border: w79 -> [w136]
    in-place-border: w74 -> [w135]
    in-place-border: w73 -> [w134]
    in-place-border: [w133] -> w66
    in-place-border: [w132] -> w62
    in-place-border: w43 -> [w129]
    in-place-border: w37 -> [w128]
    in-place-border: w36 -> [w127]
    in-place-border: w35 -> [w126]
    in-place-border: w33 -> [w125]
    in-place-border: w32 -> [w124]
    in-place-border: w31 -> [w123]
    in-place-border: w25 -> [w122]
    in-place-border: w20 -> [w121]
    in-place-border: w19 -> [w120]
    in-place-border: w18 -> [w119]
    in-place-border: w17 -> [w118]
    in-place-border: w12 -> [w117]
    in-place-border: w12 -> [w116]
    in-place-border: w7 -> [w115]
    in-place-border: w1 -> [w114]
    n43 = in-place-dvr #1("AlliGator IV DVR in") -> (w131:T14)  [unwired: 1 out]
    n44 = in-place {
      in-place-border: w145 -> [w215]
      in-place-border: w144 -> [w214]
      in-place-border: w143 -> [w213]
      in-place-border: w142 -> [w212]
      in-place-border: [w211] -> w141
      in-place-border: [w210] -> w140
      in-place-border: w139 -> [w209]
      in-place-border: w138 -> [w208]
      in-place-border: w137 -> [w207]
      in-place-border: w136 -> [w206]
      in-place-border: w135 -> [w205]
      in-place-border: w134 -> [w156]
      in-place-border: [w204] -> w133
      in-place-border: [w191] -> w132
      in-place-border: w129 -> [w192]
      in-place-border: w128 -> [w190]
      in-place-border: w127 -> [w189]
      in-place-border: w126 -> [w188]
      in-place-border: w125 -> [w162]
      in-place-border: w124 -> [w187]
      in-place-border: w123 -> [w186]
      in-place-border: w122 -> [w183]
      in-place-border: w121 -> [w175]
      in-place-border: w120 -> [w174]
      in-place-border: w119 -> [w173]
      in-place-border: w118 -> [w172]
      in-place-border: w117 -> [w164]
      in-place-border: w116 -> [w165]
      in-place-border: w115 -> [w158]
      in-place-border: w114 -> [w146]
      # "used to be [[Sum Image]]"
      # "parse formula only once"
      # "1. Gets a temp image to\nbuild the overlay"
      n45 = in-place-cluster #2(w131) -> ("[[CSG Phasors]]"=w194:csg[][], "[[Valid Pixel?]]"=w193:bool[][], "Displayed Image"=w154:T1)  [unwired: 5 out]
      n46 = call "Alligator Variables Storage.vi"("AlliGator Variable"=AlliGator_Variables_List."X_Source Image Palette Information" ("Alligator Variable"), "Error In"=w156) -> ("Error Out"=w181:errorcluster, "Data out"=w180:variant)  [unwired: 7 in, 1 out]
      n47 = Variant To Data(error in=w181, type=T9 {"Palette Name [# Colors,int?,inv?]"="", "Palette Type"=0, "Palette Colors"=[], "Interpolate?"=FALSE} ("Image Display Palette Information"), Variant=w180) -> (data=w178:T9, error out=w176:errorcluster)
      n48 = Bundle By Name(cluster=cluster{"Min Value":dbl, "Max Value":dbl} {"Min Value"=nan, "Max Value"=nan} ("Image Display Range"), "Max Value"=w175, "Min Value"=w174) -> (w147:cluster{"Min Value":dbl, "Max Value":dbl})
      n49 = call "IMAQ ImageToArray"("error in (no error)"=w156, "Image"=w154) -> ("Image Pixels (Float)"=w157:sgl[][], "error out"=w155:errorcluster)  [unwired: 2 in, 3 out]
      n50 = call "Image Display Get Pixel Color Information.vi"("Image High Color"=w173, "Image Low Color"=w172, "Error In"=w176, "Image Display Range"=w147, "Image Display Palette Information"=w178) -> ("Error Out"=w169:errorcluster, "Image Scale Factor (256 colors)"=w170:sgl, "1D Color Array"=w171:cluster{"Red":u8, "Green":u8, "Blue":u8}[])  [unwired: 3 in, 1 out]
      n51 = call "IMAQ IntegerToColorValue"("error in (no error)"=w169, "U32 value"=w213) -> ("error out"=w167:errorcluster, "Color Value"=w202:T50)  [unwired: 3 in, 2 out]
      n52 = call "IMAQ IntegerToColorValue"("error in (no error)"=w169, "U32 value"=w214) -> ("error out"=w168:errorcluster, "Color Value"=w203:T50)  [unwired: 3 in, 2 out]
      n53 = call "Create Same Type Image.vi"("error in (no error)"=w156, "Name in"="TempPhasorRatioMapOverlay", "Image Src"=w209) -> ("error out"=w198:errorcluster, "Image Dst"=w200:T1)  [unwired: 6 in, 1 out]
      n54 = call "IMAQ Clear Overlay"("error in (no error)"=w198, "Image"=w200) -> ("error out"=w197:errorcluster, "Image Out"=w199:T1)  [unwired: 8 in]
      n55 = call <vilib>:"Clear Errors.vi"("error in (no error)"=w197, "specific error code to clear (0: all)"=w208) -> ("error out"=w196:errorcluster)  [unwired: 4 in, 1 out]
      n56 = Merge Errors(w155, w196, w168, w167) -> (w161:errorcluster)
      n57 = case shown="\"User-Defined Quantity\"" w162 {
        tunnel: w164 -> [_ w434]
        tunnel: [w429 w433] -> w160
        tunnel: w161 -> [w429 w430]
        frame "Phasor Ratio (f1 or a1)", Default {
        }
        frame "User-Defined Quantity" {
          n58 = call "AlliGator Computer User-defined Quantity.vi"("Init (F)"=TRUE, "Error In"=w430, "Formula"=w434, "Basic Quantities"=sgl[] []) -> ("Error Out"=w433:errorcluster)  [unwired: 6 in, 1 out]
        }
      }
      n59 = call "High Resolution Timing.vi"("Error In"=w160) -> ("relative seconds"=w201:dbl, "Error Out"=w159:errorcluster)  [unwired: 16 in, 1 out]
      n60 = call "AlliGator Phasor Frequency.vi"() -> ("Phasor Frequency"=w163:dbl[unit])
      n61 = call "Logical Processors Used.vi"() -> ("# Logical Processor Used"=w152:i32)  [unwired: 6 in]
      n62 = for "For Loop on V lines" {
        tunnel: w194 -> [w250] mode=indexing
        tunnel: w203 -> [w249]
        tunnel: w202 -> [w248]
        tunnel: w215 -> [w247]
        tunnel: w212 -> [w246]
        tunnel: w201 -> [w244]
        tunnel: [w244] -> w204
        tunnel: w207 -> [w243]
        tunnel: w206 -> [w242]
        tunnel: w205 -> [w241]
        tunnel: w199 -> [w253]
        tunnel: [w251] -> w150
        tunnel: [w240] -> w211 mode=indexing
        tunnel: w161 -> [w252]
        tunnel: [w239] -> w153 mode=concatenating
        tunnel: w193 -> [w238] mode=indexing
        tunnel: w192 -> [w237]
        tunnel: [w236] -> w185 mode=indexing
        tunnel: w190 -> [w235]
        tunnel: w189 -> [w234]
        tunnel: w188 -> [w233]
        tunnel: w162 -> [w232]
        tunnel: w187 -> [w231]
        tunnel: w186 -> [w230]
        tunnel: w183 -> [w229]
        tunnel: [w228] -> w184 mode=indexing
        tunnel: w157 -> [w227]
        workers-P: w152 -> [_]
        tunnel: w171 -> [w226]
        tunnel: w170 -> [w225]
        tunnel: [w224] -> w149 mode=indexing
        tunnel: [w223] -> w148
        tunnel: w164 -> [w222]
        tunnel: [w221] -> w166 mode=indexing
        tunnel: w159 -> [w220]
        tunnel: w163 -> [w219]
        tunnel: w158 -> [w218]
        tunnel: w147 -> [w217]
        tunnel: w146 -> [w216]
        i -> [w254]
        w223 = "Phasor Ratio Map Overlay" ("Group")
        # "y"
        n63 = for "For Loop on H columns" {
          tunnel: w254 -> [w283]
          tunnel: w223 -> [w292]
          tunnel: w250 -> [w287] mode=indexing
          tunnel: w249 -> [w286]
          tunnel: w248 -> [w285]
          tunnel: w247 -> [w288]
          tunnel: w246 -> [w284]
          tunnel: w243 -> [w281]
          tunnel: w242 -> [w280]
          tunnel: w241 -> [w279]
          tunnel: w253 -> [w293]
          tunnel: [w290] -> w251
          tunnel: w252 -> [w291]
          tunnel: [w289] -> w239 mode=indexing
          tunnel: [w277] -> w245 mode=indexing if=w278
          tunnel: w238 -> [w275] mode=indexing
          tunnel: w237 -> [w276]
          tunnel: [w274] -> w236 mode=indexing
          tunnel: w235 -> [w273]
          tunnel: w234 -> [w272]
          tunnel: w233 -> [w271]
          tunnel: w232 -> [w270]
          tunnel: w231 -> [w269]
          tunnel: w230 -> [w268]
          tunnel: w229 -> [w267]
          tunnel: [w266] -> w228 mode=indexing
          tunnel: w227 -> [w265]
          tunnel: w226 -> [w264]
          tunnel: w225 -> [w263]
          tunnel: [w262] -> w224 mode=indexing
          tunnel: w222 -> [w261]
          tunnel: [w260] -> w221 mode=indexing
          tunnel: w220 -> [w259]
          tunnel: w219 -> [w258]
          tunnel: w218 -> [w257]
          tunnel: w217 -> [w256]
          tunnel: w216 -> [w255]
          i -> [w282]
          # "x"
          n64 = case shown="True" w275 {
            tunnel: w293 -> [w297 w342]
            tunnel: w292 -> [_ w341]
            tunnel: w291 -> [w296 w340]
            tunnel: [w297 w338] -> w290
            tunnel: [w296 w337] -> w289
            tunnel: w288 -> [_ w335]
            tunnel: w287 -> [_ w307]
            tunnel: w286 -> [_ w334]
            tunnel: w285 -> [_ w333]
            tunnel: w284 -> [_ w332]
            tunnel: w283 -> [_ w322]
            tunnel: w282 -> [_ w323]
            tunnel: w281 -> [_ w331]
            tunnel: w280 -> [_ w330]
            tunnel: w279 -> [_ w329]
            tunnel: [_ w327] -> w278
            tunnel: [_ 1] -> w277
            tunnel: w276 -> [_ w325]
            tunnel: [w294 w306] -> w274
            tunnel: w273 -> [_ w321]
            tunnel: w272 -> [_ w309]
            tunnel: w271 -> [_ w320]
            tunnel: w270 -> [_ w319]
            tunnel: w269 -> [_ w314]
            tunnel: w268 -> [_ w313]
            tunnel: w267 -> [_ w315]
            tunnel: [w294 w305] -> w266
            tunnel: w265 -> [_ w318]
            tunnel: w264 -> [_ w303]
            tunnel: w263 -> [_ w317]
            tunnel: [u32 16777216 ("Reference 1") w316] -> w262
            tunnel: w261 -> [_ w312]
            tunnel: [w294 w311] -> w260
            tunnel: w259 -> [_ w310]
            tunnel: w258 -> [_ w308]
            tunnel: w257 -> [_ w301]
            tunnel: w256 -> [_ w299]
            tunnel: w255 -> [_ w298]
            frame False {
              w294 = sgl nan
            }
            frame True {
              n65 = call "Phasor Get Phasor Ratio.vi"("z"=w307, "Error In"=w310, "Reference Phasor 2"=w320, "Reference Phasor 1"=w309) -> ("Error Out"=w304:errorcluster, "Phasor Ratio (f1)"=w306:dbl)  [unwired: 5 in, 1 out]
              n66 = case shown="\"User-Defined Quantity\"" w319 {
                tunnel: [w382 w389 w409] -> w311
                tunnel: w315 -> [w383 w390 w403]
                tunnel: w314 -> [w386 w393 w400]
                tunnel: w313 -> [w385 w392 w399]
                tunnel: w306 -> [w384 w391 w401]
                tunnel: w312 -> [_ _ w408]
                tunnel: w304 -> [w379 w388 w397]
                tunnel: w308 -> [_ _ w402]
                tunnel: w307 -> [_ _ w398]
                tunnel: [w380 w389 w406] -> w305
                tunnel: [w378 w387 w396] -> w302
                tunnel: w301 -> [_ _ w395]
                frame "Phasor Ratio (f1 or a1)", Default {
                  # "f1 or a1 depending on average lifetime option"
                  n67 = call "Phasor Convert Ratio to Amplitude Ratio & Average Lifetime.vi"("Compute Amplitude Ratio"=w383, "error in (no error)"=w379, "Reference Lifetime 2"=w385, "Reference Lifetime 1"=w386, "Phasor Ratio (f1)"=w384) -> ("error out"=w378:errorcluster, "Average Lifetime"=w381:dbl[unit], "Phasor/Amplitude Ratio"=w382:dbl)  [unwired: 2 in, 2 out]
                  n68 = node(w381) -> (w380:dbl)
                }
                frame "Average Lifetime (<tau>_i or <tau>_a))" {
                  # "<tau>_i or <tau>_a depending on average lifetime option"
                  n69 = call "Phasor Convert Ratio to Amplitude Ratio & Average Lifetime.vi"("Compute Amplitude Ratio"=w390, "error in (no error)"=w388, "Reference Lifetime 2"=w392, "Reference Lifetime 1"=w393, "Phasor Ratio (f1)"=w391) -> ("error out"=w387:errorcluster, "Average Lifetime"=w394:dbl[unit])  [unwired: 2 in, 3 out]
                  n70 = node(w394) -> (w389:dbl)
                }
                frame "User-Defined Quantity" {
                  n71 = call "AlliGator Compute Basic Quantities.vi"("Phasor Ratio (f1)"=w401, "Data Information"=w395, "Reference Lifetime 1"=w400, "Reference Lifetime 2"=w399, "Complex Phasor"=w398, "error in (no error)"=w397, "Phasor Frequency"=w402, "Compute Amplitude Ratio"=w403) -> ("Average Lifetime"=w406:dbl, "Basic Quantities"=w405:dbl[], "error out"=w404:errorcluster)  [unwired: 5 in]
                  n72 = call "AlliGator Computer User-defined Quantity.vi"("Init (F)"=FALSE, "Error In"=w404, "Formula"=w408, "Basic Quantities"=w405) -> ("Error Out"=w396:errorcluster, "User-defined Quantity"=w409:sgl)  [unwired: 6 in]
                }
              }
              n73 = Bundle By Name(cluster=w325, "Complex Phasor"=w307, "Phasor Ratio"=w306, "Mapped Quantity"=w311) -> (w324:T7)
              n74 = case shown="\"Use Custom Map\"" w330 {
                tunnel: w335 -> [w415 w425]
                tunnel: [w419 w428] -> w336
                tunnel: w334 -> [w414 _]
                tunnel: w333 -> [w413 _]
                tunnel: [w418 w427] -> w328
                tunnel: w332 -> [w416 w424]
                tunnel: w329 -> [_ w422]
                tunnel: w324 -> [w417 w426]
                tunnel: w321 -> [w412 w423]
                tunnel: w302 -> [w411 w421]
                tunnel: [w410 w420] -> w300
                frame "Interpolate Reference Colors", Default {
                  n75 = call "AlliGator Get Phasor Ratio Interpolated Color v2.vi"("Color 2"=w413, "Color 1"=w414, "Color Fading?"=w416, "Error In"=w411, "Phasor Ratio/Average Lifetime Display Range"=w412, "-d_0"=w415, "Phasor Ratio Data"=w417) -> ("Error Out"=w410:errorcluster, "Transparent?"=w418:bool, "Overlay Color"=w419:T50)  [unwired: 2 in]
                }
                frame "Use Custom Map" {
                  n76 = call "AlliGator Get Phasor Ratio Map Color v2.vi"("Image Display Palette Information"=w422, "Color Fading?"=w424, "Error In"=w421, "Phasor Ratio Display Range"=w423, "-d_0"=w425, "Phasor Ratio Data"=w426) -> ("Error Out"=w420:errorcluster, "Transparent?"=w427:bool, "Overlay Color"=w428:T50)  [unwired: 3 in]
                }
              }
              n77 = case shown="False" w328 {
                tunnel: w342 -> [w356 w376]
                tunnel: w336 -> [w358 _]
                tunnel: w341 -> [_ _]
                tunnel: w340 -> [w357 w377]
                tunnel: [w347 w377] -> w339
                tunnel: [w352 w376] -> w338
                tunnel: w323 -> [w355 _]
                tunnel: w322 -> [w354 _]
                tunnel: w331 -> [w353 _]
                tunnel: w318 -> [w351 _]
                tunnel: w303 -> [w350 _]
                tunnel: w317 -> [w349 _]
                tunnel: [w348 u32 16777216 ("Reference 1")] -> w316
                tunnel: w300 -> [_ _]
                tunnel: w299 -> [w344 _]
                tunnel: w298 -> [w343 _]
                frame False {
                  # "Not transparent"
                  n78 = case shown="True" w353 {
                    tunnel: [w360 w368] -> w345
                    tunnel: w358 -> [w361 w365]
                    tunnel: [w361 w369] -> w346
                    tunnel: w357 -> [w360 w367]
                    tunnel: w356 -> [w359 w372]
                    tunnel: w355 -> [_ w374]
                    tunnel: w354 -> [_ w373]
                    tunnel: [w359 w372] -> w352
                    tunnel: w351 -> [_ w371]
                    tunnel: w350 -> [_ w366]
                    tunnel: w349 -> [_ w363]
                    tunnel: w344 -> [_ w364]
                    tunnel: w343 -> [_ w362]
                    frame False {
                      # "Display overlay color as is"
                    }
                    frame True {
                      # "Use Image Brightness"
                      n79 = Index Array(array=w371, index (row)=w373, index (col)=w374) -> (element=w370:sgl)
                      n80 = call "Blend Overlay Color with Background.vi"("Overlay Color Value"=w365, "Image Scale Factor"=w363, "Blend Overlay with Background"=w362, "error in (no error)"=w367, "Image Display Range"=w364, "Image Color Array"=w366, "Pixel Value"=w370) -> ("error out"=w368:errorcluster, "Scaled/Blended Overlay Color Value"=w369:T50)  [unwired: 3 in]
                    }
                  }
                  n81 = call "IMAQ ColorValueToInteger"("error in (no error)"=w345, "Color Value"=w346) -> ("error out"=w347:errorcluster, "U32 value"=w348:u32)  [unwired: 3 in, 2 out]
                }
                frame True {
                  # "Transparent overlay"
                }
              }
              n82 = call "Clear Error.vi"("Error In"=w339) -> ("no Error Out"=w337:errorcluster)  [unwired: 8 in]
              n83 = Not(x=w328) -> (.not. x?=w327:bool)
            }
          }
        }
        n84 = Add Array Elements(numeric array=w245) -> (sum=w240:i32)
      }
      n85 = Merge Errors(w153) -> (w151:errorcluster)
      n86 = call "IMAQ Overlay Bitmap"("Group"=w148, "error in (no error)"=w151, "Bitmap"=w149, "Image"=w150) -> ("error out"=w191:errorcluster, "Image Out"=w210:T1)  [unwired: 6 in]
      n87 = in-place-cluster #2("[[CSG Phasors]]"=w194, "[[Valid Pixel?]]"=w193, "[[Phasor Ratios]]"=w185, "[[Average Lifetimes]]"=w184, "[[User-defined Quantities]]"=w166, "User-defined Quantity"=w165, "Amplitude Weighted Average Lifetime"=w183, "Displayed Image"=w154) -> (w130:T14)
    }
    n88 = in-place-dvr #1(w130) -> (→"AlliGator IV DVR out":refnum<data-value>, w51:errorcluster)
  }
  n89 = Add Array Elements(numeric array=w93) -> (sum=→"# Overlay Pixels":i32)
  n90 = Merge Errors(w51, w62) -> (w57:errorcluster)
  n91 = call "High Resolution Timing.vi"("relative seconds (NaN)"=w66, "Error In"=w57) -> ("relative seconds"=w64:dbl, "elapsed (relative) seconds"=→"Overlay Compute (s)":dbl, "Error Out"=w63:errorcluster)  [unwired: 15 in]
  n92 = call "IMAQ Clear Overlay"("error in (no error)"=w63, "Image"="Source Image Display") -> ("error out"=w89:errorcluster, "Image Out"=w92:T1)  [unwired: 8 in]
  n93 = call <vilib>:"Clear Errors.vi"("error in (no error)"=w89, "specific error code to clear (0: all)"=w88) -> ("error out"=w56:errorcluster)  [unwired: 4 in, 1 out]
  n94 = call "High Resolution Timing.vi"("relative seconds (NaN)"=w64, "Error In"=w56) -> ("relative seconds"=w60:dbl, "elapsed (relative) seconds"=→"Overlay Erase (s)":dbl, "Error Out"=w55:errorcluster)  [unwired: 15 in]
  n95 = call "IMAQ Copy Overlay"("error in (no error)"=w55, "Image Dst"=w92, "Image Src"=w90) -> ("error out"=w54:errorcluster, "Image Dst Out"=→"Source Image Display out":T1)  [unwired: 7 in]
  n96 = call "High Resolution Timing.vi"("relative seconds (NaN)"=w60, "Error In"=w54) -> ("elapsed (relative) seconds"=→"Overlay Copy (s)":dbl, "Error Out"=→"Error Out":errorcluster)  [unwired: 15 in, 1 out]
